vi "ui_DataLog Query Tag Configuration.vi"(7 "info in":T3 {"logging parameters" format="%.2e"; "precision" items=["0", "1", "2", "3", "4", "5", "6", "7", "8", "9", "10", "11", "12", "13", "14", "15", "16", "17"]; "limit delay" format="%.2e"; "deadband" format="%.2e"}) -> (4 "OKed?":bool, 8 "info out":T3 {"logging parameters" format="%.2e"; "precision" items=["0", "1", "2", "3", "4", "5", "6", "7", "8", "9", "10", "11", "12", "13", "14", "15", "16", "17"]; "limit delay" format="%.2e"; "deadband" format="%.2e"})   [LabVIEW 2012]
doc: "This dialog allows the modifiable tag properties to be configured or reconfigured. This is not the sum of all tag properties. Other properties exists that are set programatically, as meta tags, or at creation time only."
uses:
  typedefs/t_DataLog Logging Algorithms.ctl
  typedefs/t_DataLog Numerical Format.ctl
  typedefs/clusters/t_DataLog Tag Config.ctl
  typedefs/t_DataLog Temporal Types.ctl
  typedefs/t_DataLog Value Types.ctl
  typedefs/t_DataLog Query Tag Configuration States.ctl
panel:
  in  "undefine":bool
  in  "update period (ms)":u16=10 min=10
  in  "update":bool
  in  "clear":bool
  in  "logging parameters":dbl[](array[numeric])
  in  "precision":u8(ring) items=["0", "1", "2", "3", "4", "5", "6", "7", "8", "9", "10", "11", "12", "13", "14", "15", "16", "17"]
  in  "format":T1
  out "format example":dbl format="%.2f"
  in  "min capacity":i32
  out "unit":string
  in  "limit delay (s)":dbl min=0.0 format="%.2f"
  in  "logging algorithm":T2
  in  "description":string
  in  "deadband":dbl min=0.0 format="%.4e"
  in  "expression":string
  in  "cancel":bool
  in  "OK":bool
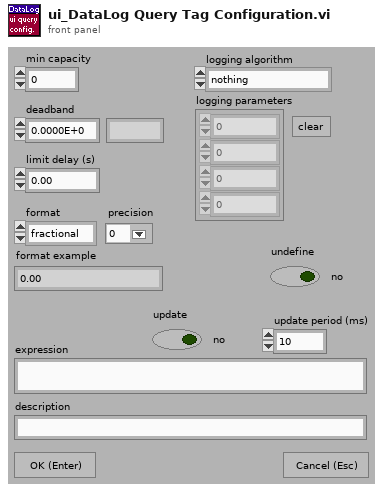
[diagram p1: front panel]
types:
  T1 = typedef "t_DataLog Numerical Format.ctl" = enum8{"fractional", "exponential", "engineering"}
  T2 = typedef "t_DataLog Logging Algorithms.ctl" = enum16{"nothing", "changes", "everything", "every Nth", "time threshold", "value threshold + prior", "t or v threshold", "t or v threshold + prior"}
  T3 = typedef "t_DataLog Tag Config.ctl" = cluster{"name":string, "unit":string, "temporal":T4, "value":T5, "index":i32, "capacity":i32, "is meta?":bool, "mincapacity":i32, "deadband":dbl, "limit delay":dbl, "format":T1, "precision":u8, "undefine":bool, "update":bool, "update period":u16, "expression":string, "description":string, "logging algorithm":T2, "logging parameters":dbl[]}
  T4 = typedef "t_DataLog Temporal Types.ctl" = enum16{"set&hold", "sample", "event"}
  T5 = typedef "t_DataLog Value Types.ctl" = enum16{"number", "string"}
  T6 = typedef "t_DataLog Query Tag Configuration States.ctl" = enum16{"empty queue", "apply format", "initialize", "stop"}
  T7 = typedef "eventvkey.ctl" = enum16{"ASCII", "Enter", "Return", "Shift", "Ctrl", "Alt", "Cmd", "Opt", "Caps", "NumLock", "Clear", "Break", "Up", "Down", "Left", "Right", "Insert", "Delete", "Home", "End", "PageUp", "PageDown", "Escape", "Help", "Pause", "ScrollLock", "F1", "F2", "F3", "F4", "F5", "F6", "F7", "F8", "F9", "F10", "F11", "F12", "F13", "F14", "F15", "F16", "F17", "F18", "F19", "F20", "F21", "F22", "F23", "F24", "Play", "VolumeUp", "VolumeDown", "Mute", "Two Byte Char"}
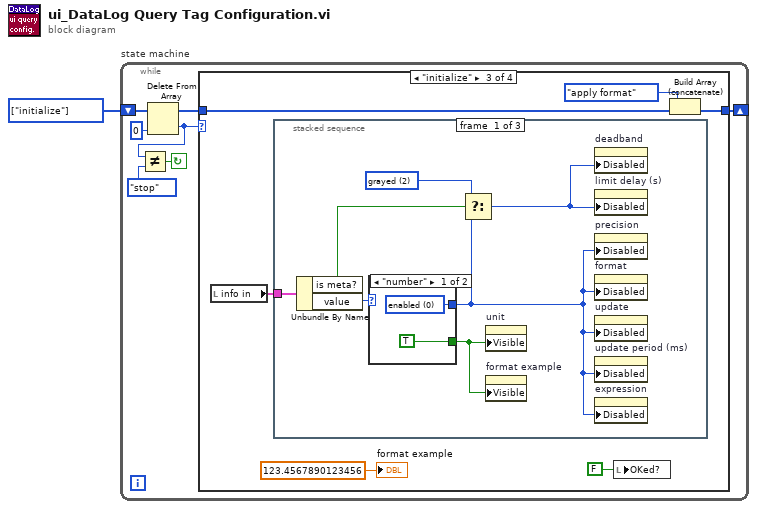
[diagram p0: block diagram]
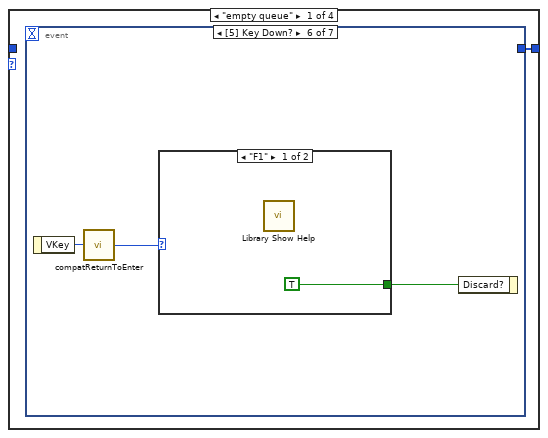
[diagram p2: hidden frame]
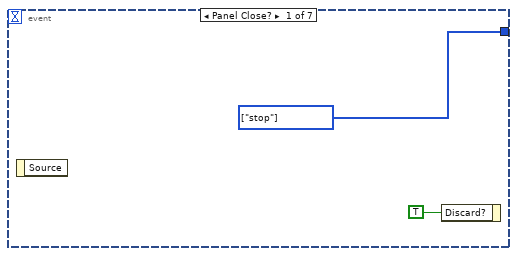
[diagram p3: hidden frame]
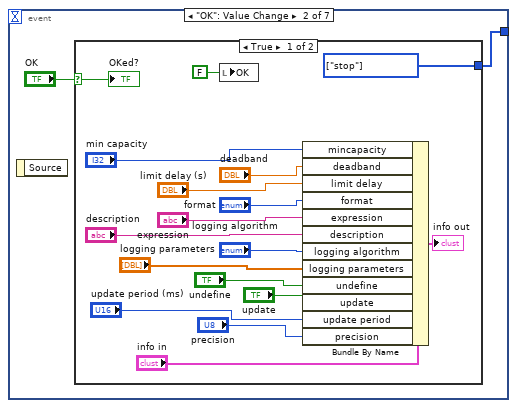
[diagram p4: hidden frame]
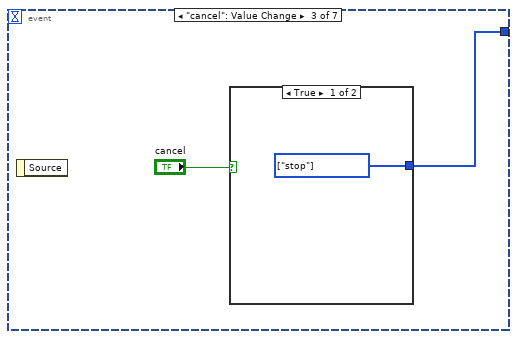
[diagram p6: hidden frame]
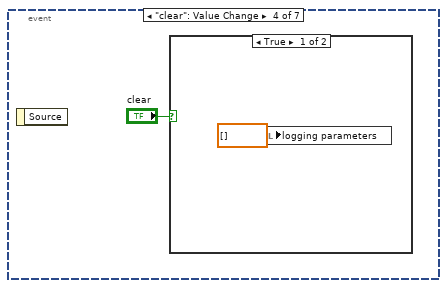
[diagram p8: hidden frame]
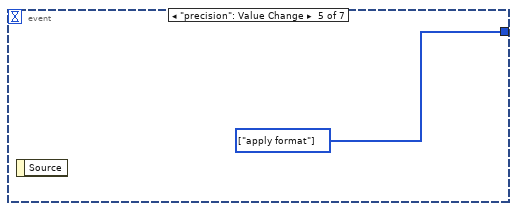
[diagram p10: hidden frame]
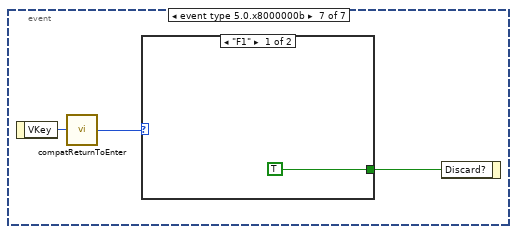
[diagram p12: hidden frame]
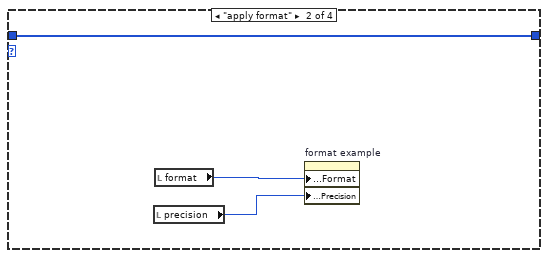
[diagram p14: hidden frame]
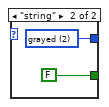
[diagram p15: hidden frame]
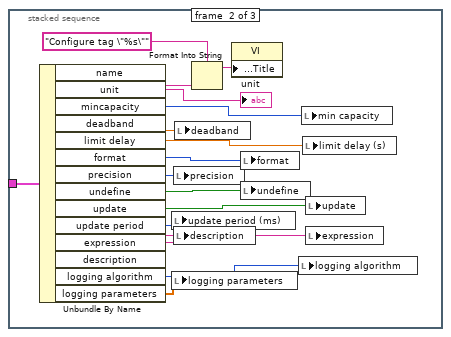
[diagram p16: hidden frame]
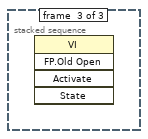
[diagram p17: hidden frame]
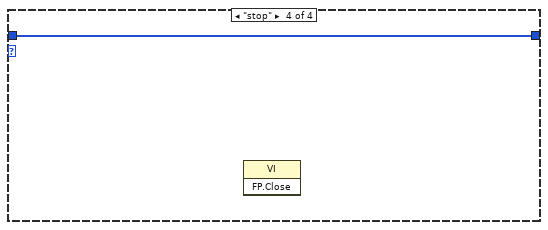
[diagram p18: hidden frame]
diagram:
  w1 = T6[] [enum."initialize"] items=["empty queue", "apply format", "initialize", "stop"] ("Array Constant")
  n1 = while "state machine" {
    shift-left: w1 -> [w5]
    shift-right: [w8] -> _
    stop <- w7 continue-if-true
    n2 = Delete From Array(array=w5, index=0) -> (deleted portion=w3:T6, array with subset deleted=w4:T6[])  [unwired: 1 in]
    n3 = Not Equal?(x=w3, y=t_DataLog_Query_Tag_Configuration_States."stop" ("states")) -> (x != y?=w7:bool)
    n4 = case "Case" shown="\"initialize\"" w3 {
      tunnel: [w9 w47 w50 w82] -> w8
      tunnel: w4 -> [_ w47 w53 w82]
      frame "empty queue" {
        n5 = event shown="[5] Key Down?" {
          selector: _ -> [_ _ _ _ _ _ _]
          dyn-events: _ -> [_ _ _ _ _ _ _]
          timeout: _ -> [_ _ _ _ _ _ _]
          tunnel: [w11 w13 w32 _ w36 _ _] -> w9
          event Panel Close? {
            w11 = T6[] [enum."stop"] items=["empty queue", "apply format", "initialize", "stop"] ("Array Constant")
            n6 = event-data() -> ()  [unwired: 1 in, 1 out]
            n7 = event-data("Discard?"=TRUE) -> ()  [unwired: 1 in, 1 out]
          }
          event "OK": Value Change {
            n8 = event-data() -> ()  [unwired: 1 in, 1 out]
            n9 = case shown="True" "OK" {
              selector: "OK" -> [w29 _]
              tunnel: [w30 _] -> w13
              frame True {
                w30 = T6[] [enum."stop"] items=["empty queue", "apply format", "initialize", "stop"] ("Array Constant")
                n10 = local write "OK"(FALSE ("OK")) -> ()
                n11 = Bundle By Name(cluster="info in", "mincapacity"="min capacity", "deadband"="deadband", "limit delay"="limit delay (s)", "format"="format", "expression"="expression", "description"="description", "logging algorithm"="logging algorithm", "logging parameters"="logging parameters", "undefine"="undefine", "update"="update", "update period"="update period (ms)", "precision"="precision") -> (→"info out":T3)
                "OKed?" <- w29
              }
              frame False {
              }
            }
          }
          event "cancel": Value Change {
            n12 = event-data() -> ()  [unwired: 1 in, 1 out]
            n13 = case shown="True" "cancel" {
              tunnel: [w33 _] -> w32
              frame True {
                w33 = T6[] [enum."stop"] items=["empty queue", "apply format", "initialize", "stop"] ("Array Constant")
              }
              frame False {
              }
            }
          }
          event "clear": Value Change {
            n14 = event-data() -> ()  [unwired: 1 in, 1 out]
            n15 = case shown="True" "clear" {
              frame True {
                n16 = local write "logging parameters"(dbl[] [] ("logging parameters")) -> ()
              }
              frame False {
              }
            }
          }
          event "precision": Value Change {
            w36 = T6[] [enum."apply format"] items=["empty queue", "apply format", "initialize", "stop"] ("Array Constant")
            n17 = event-data() -> ()  [unwired: 1 in, 1 out]
          }
          event Key Down? {
            n18 = event-data() -> ("VKey"=w37:T7)  [unwired: 1 in]
            n19 = call <vilib>:"compatReturnToEnter.vi"("VKey"=w37) -> ("VKey"=w38:T7)
            n20 = case shown="\"F1\"" w38 {
              tunnel: [TRUE _] -> w39
              frame "F1" {
                n21 = call "Library Show Help.vi"() -> ()  [unwired: 1 in]
              }
              frame Default {
              }
            }
            n22 = event-data("Discard?"=w39) -> ()  [unwired: 1 in, 1 out]
          }
          event event type 5.0.x8000000b {
            n23 = event-data() -> ("VKey"=w41:T7)  [unwired: 1 in]
            n24 = call <vilib>:"compatReturnToEnter.vi"("VKey"=w41) -> ("VKey"=w42:T7)
            n25 = case shown="\"F1\"" w42 {
              tunnel: [TRUE _] -> w43
              frame "F1" {
              }
              frame Default {
              }
            }
            n26 = event-data("Discard?"=w43) -> ()  [unwired: 1 in, 1 out]
          }
        }
      }
      frame "apply format" {
        n27 = local read "precision"() -> (w45:u8)
        n28 = local read "format"() -> (w46:T1)
        n29 = property on="format example" class="DigNum (strict)"("Display Format:Format"=w46, "Display Format:Precision"=w45) -> ()  [unwired: 2 in, 2 out]
      }
      frame "initialize" {
        n30 = local read "info in"() -> (w51:T3)
        n31 = stacked-sequence {
          tunnel: w51 -> [w60 w81 _]
          frame #0 {
            w58 = u8 2 items=["enabled", "disabled", "grayed"] ("disabled state")
            n32 = Unbundle By Name(w60) -> ("is meta?"=w59:bool, "value"=w56:T5)
            n33 = case shown="\"number\"" w56 {
              tunnel: [w62 w64] -> w55
              tunnel: [TRUE FALSE] -> w54
              frame "number" {
                w62 = u8 0 items=["enabled", "disabled", "grayed"] ("disabled state")
              }
              frame "string" {
                w64 = u8 2 items=["enabled", "disabled", "grayed"] ("disabled state")
              }
            }
            n34 = Select(t=w58, s=w59, f=w55) -> (s? t:f=w57:u8)
            n35 = property on="unit" class="Str"("Visible"=w54) -> ()  [unwired: 2 in, 2 out]
            n36 = property on="format example" class="DigNum (strict)"("Visible"=w54) -> ()  [unwired: 2 in, 2 out]
            n37 = property on="deadband" class="DigNum (strict)"("Disabled"=w57) -> ()  [unwired: 2 in, 2 out]
            n38 = property on="limit delay (s)" class="DigNum (strict)"("Disabled"=w57) -> ()  [unwired: 2 in, 2 out]
            n39 = property on="precision" class="Ring (strict)"("Disabled"=w55) -> ()  [unwired: 2 in, 2 out]
            n40 = property on="format" class="Enum (strict)"("Disabled"=w55) -> ()  [unwired: 2 in, 2 out]
            n41 = property on="update" class="Bool (strict)"("Disabled"=w55) -> ()  [unwired: 2 in, 2 out]
            n42 = property on="update period (ms)" class="DigNum (strict)"("Disabled"=w55) -> ()  [unwired: 2 in, 2 out]
            n43 = property on="expression" class="Str"("Disabled"=w55) -> ()  [unwired: 2 in, 2 out]
          }
          frame #1 {
            n44 = Unbundle By Name(w81) -> ("name"=w72:string, "unit"=→"unit":string, "mincapacity"=w73:i32, "deadband"=w75:dbl, "limit delay"=w76:dbl, "format"=w69:T1, "precision"=w68:u8, "undefine"=w65:bool, "update"=w67:bool, "update period"=w66:u16, "expression"=w77:string, "description"=w78:string, "logging algorithm"=w79:T2, "logging parameters"=w80:dbl[])
            n45 = local write "update period (ms)"(w66) -> ()
            n46 = local write "logging parameters"(w80) -> ()
            n47 = local write "precision"(w68) -> ()
            n48 = local write "description"(w78) -> ()
            n49 = local write "deadband"(w75) -> ()
            n50 = Format Into String(format string="Configure tag \"%s\"", w72) -> (resulting string=w70:string)  [unwired: 2 in, 1 out]
            n51 = property class="VI"("Front Panel Window:Title"=w70) -> ()  [unwired: 2 in, 2 out]
            n52 = local write "format"(w69) -> ()
            n53 = local write "undefine"(w65) -> ()
            n54 = local write "logging algorithm"(w79) -> ()
            n55 = local write "min capacity"(w73) -> ()
            n56 = local write "limit delay (s)"(w76) -> ()
            n57 = local write "update"(w67) -> ()
            n58 = local write "expression"(w77) -> ()
          }
          frame #2 {
            n59 = invoke class="VI" method="FP.Old Open"() -> ()  [unwired: 5 in, 5 out]
          }
        }
        n60 = local write "OKed?"(FALSE ("OKed?")) -> ()
        n61 = Build Array (concatenate)(t_DataLog_Query_Tag_Configuration_States."apply format" ("states"), w53) -> (w50:T6[])
        "format example" <- 123.4567890123456
      }
      frame "stop" {
        n62 = invoke class="VI" method="FP.Close"() -> ()  [unwired: 3 in, 3 out]
      }
    }
  }
